vi "slowbounds.vi"(2 "HV Cluster":T2={"HV Power On/Off"=[], "Set Voltage"=[], "HV Tolerance (%)"=1.0}, 3 "Slow Cluster":T1={"Number of Slow Parameters"=0, "UTC format?"=TRUE, "Sensor Upper bounds"=[85, 1000000, 8000, 8000, 8000, 14000, 99, 33000], "Sensor Lower bounds"=[-40, 0, -8000, -8000, -8000, -14000, 0, -33000], "datanames"=[], "Descriptions"=[]}) -> (0 "Lower Bounds":dbl[](array[numeric]), 1 "Upper Bounds":dbl[](array[numeric]))   [LabVIEW 2012]
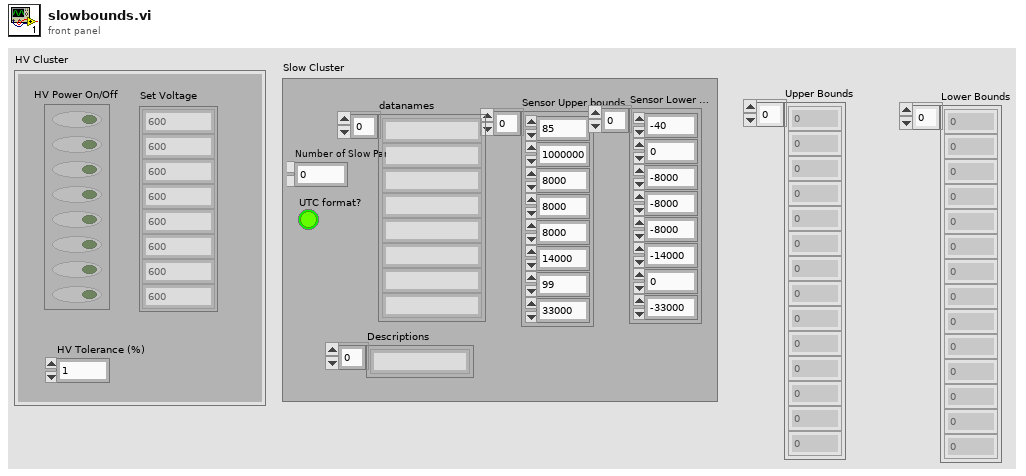
[diagram p1: front panel]
types:
  T1 = cluster{"Number of Slow Parameters":i32, "UTC format?":bool, "Sensor Upper bounds":i32[], "Sensor Lower bounds":i32[], "datanames":string[], "Descriptions":string[]}
  T2 = cluster{"HV Power On/Off":bool[], "Set Voltage":string[], "HV Tolerance (%)":dbl}
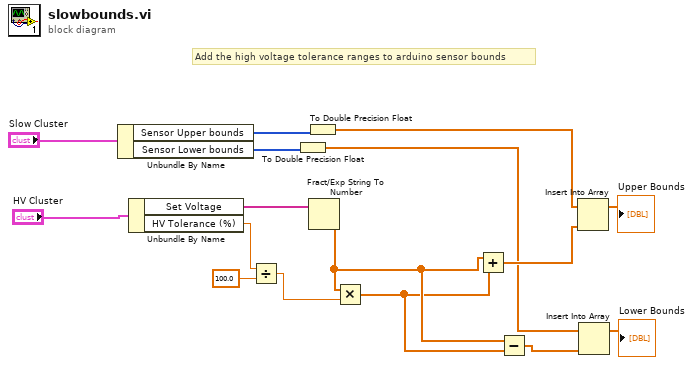
[diagram p0: block diagram]
diagram:
  # "Add the high voltage tolerance ranges to arduino sensor bounds"
  n1 = Unbundle By Name("Slow Cluster") -> ("Sensor Upper bounds"=w4:i32[], "Sensor Lower bounds"=w3:i32[])
  n2 = Unbundle By Name("HV Cluster") -> ("Set Voltage"=w14:string[], "HV Tolerance (%)"=w7:dbl)
  n3 = Divide(x=w7, y=100.0) -> (x/y=w5:dbl)
  n4 = To Double Precision Float(number=w3) -> (double precision float=w1:dbl[])
  n5 = To Double Precision Float(number=w4) -> (double precision float=w2:dbl[])
  n6 = Fract/Exp String To Number(string=w14) -> (number=w13:dbl[])  [unwired: 3 in, 1 out]
  n7 = Multiply(x=w13, y=w5) -> (x*y=w12:dbl[])
  n8 = Add(x=w13, y=w12) -> (x+y=w11:dbl[])
  n9 = Subtract(x=w13, y=w12) -> (x-y=w10:dbl[])
  n10 = Insert Into Array(array=w2, new element=w11) -> (→"Upper Bounds":dbl[])  [unwired: 1 in]
  n11 = Insert Into Array(array=w1, new element=w10) -> (→"Lower Bounds":dbl[])  [unwired: 1 in]
